vi "instrument info parser.vi"(4 "ID":string) -> (1 "Instrument Info":string[](array[string]))   [LabVIEW 2025]
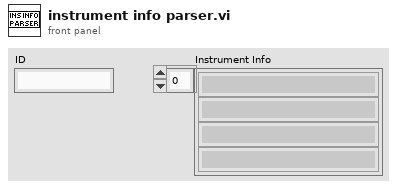
[diagram p1: front panel]
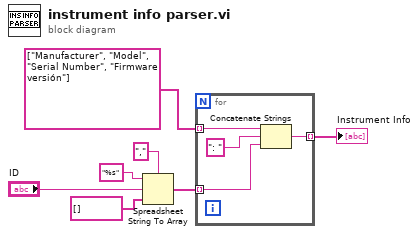
[diagram p0: block diagram]
diagram:
  n1 = Spreadsheet String To Array(delimiter (Tab)="," ("delimiter"), format string="%s", spreadsheet string="ID", array type (2D Dbl)=string[] []) -> (array=w1:string[])
  n2 = for {
    tunnel: w1 -> [w9] mode=indexing
    tunnel: string[] ["Manufacturer", "Model", "Serial Number", "Firmware versión"] -> [w11] mode=indexing
    tunnel: [w8] -> w6 mode=indexing
    n3 = Concatenate Strings(w11, ": ", w9) -> (w8:string)
  }
  "Instrument Info" <- w6
